vi "Average_ITP_curves.vi"(0 "I in":dbl[](array[numeric]), 1 "Averaged P(T) In":dbl[][](array[numeric]), 2 "Counter":i8, 5 "Averaged I(T) In":dbl[][](array[numeric]), 7 "t in":dbl[](array[numeric]), 9 "T in":dbl[](array[numeric]), 11 "Averaged dt in":dbl[][](array[numeric]), 12 "Up/Down":bool, 13 "Sample area(mm^2)":dbl, 14 "T array":dbl[](array[numeric])) -> (4 "Averaged I(B) out":dbl[][](array[numeric]), 6 "Averaged dt Out":dbl[][](array[numeric]), 8 "Averaged P(T) Out":dbl[][](array[numeric]))   [LabVIEW 2015]
uses:
  <vilib>/Analysis/baseanly.llb/Mean (DBL).vi
  <vilib>/Analysis/NI_AALBase.lvlib
  <vilib>/gmath/NI_Gmath.lvlib
panel:
  out "yi":dbl[](array[numeric]) format="%_6g"
  out "Down":cluster{"B array":dbl[], dbl[]}(graph)
  out "XY Graph 2":cluster{"B in":dbl[], "I in":dbl[]}(graph)
  out "Up":cluster{"B array":dbl[], dbl[]}(graph)
  out "subarray 2":dbl[](array[numeric])
  out "subarray":dbl[](array[numeric])
  out "Sorted array":dbl[][](array[numeric]) format="%.5f"
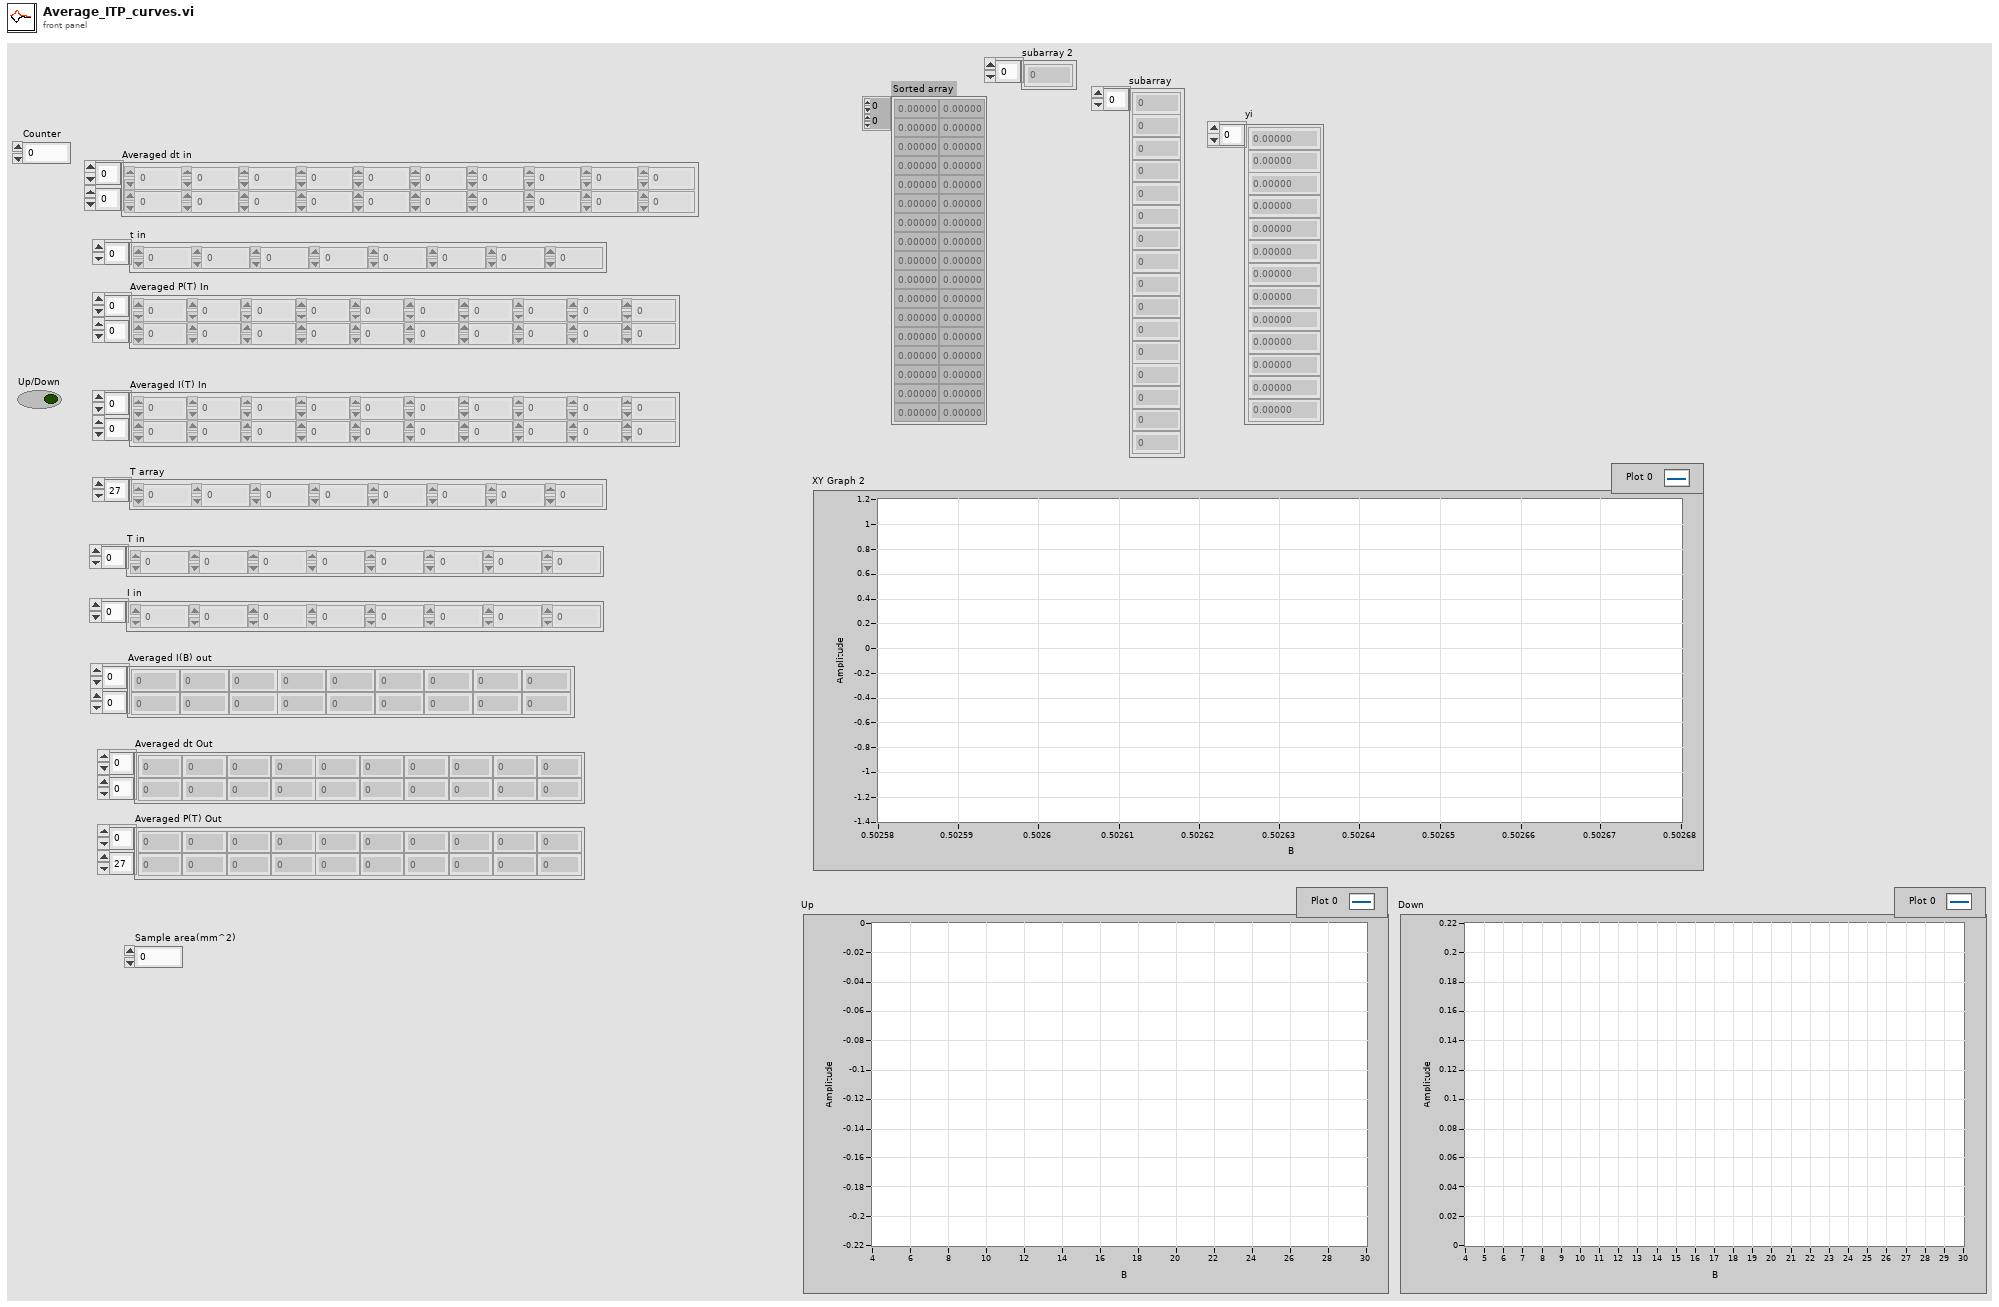
[diagram p1: front panel]
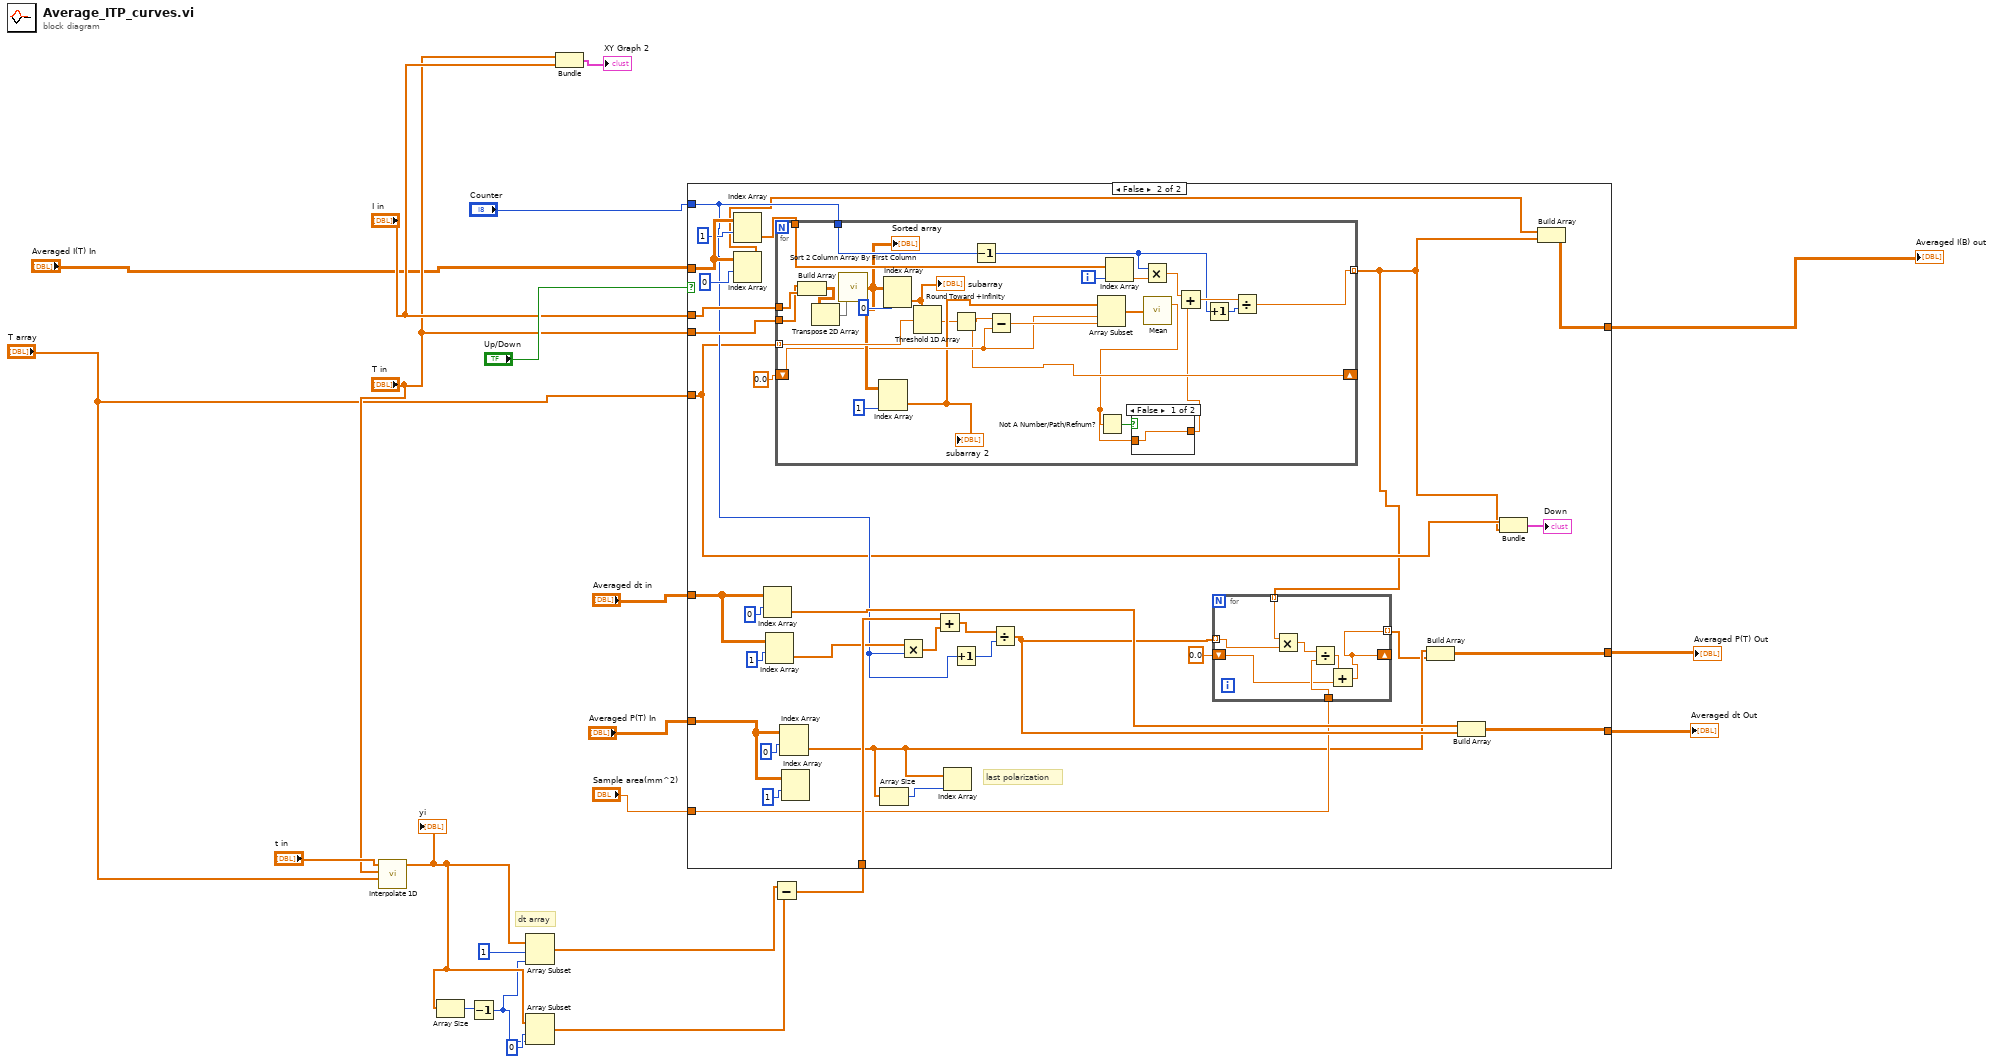
[diagram p0: block diagram]
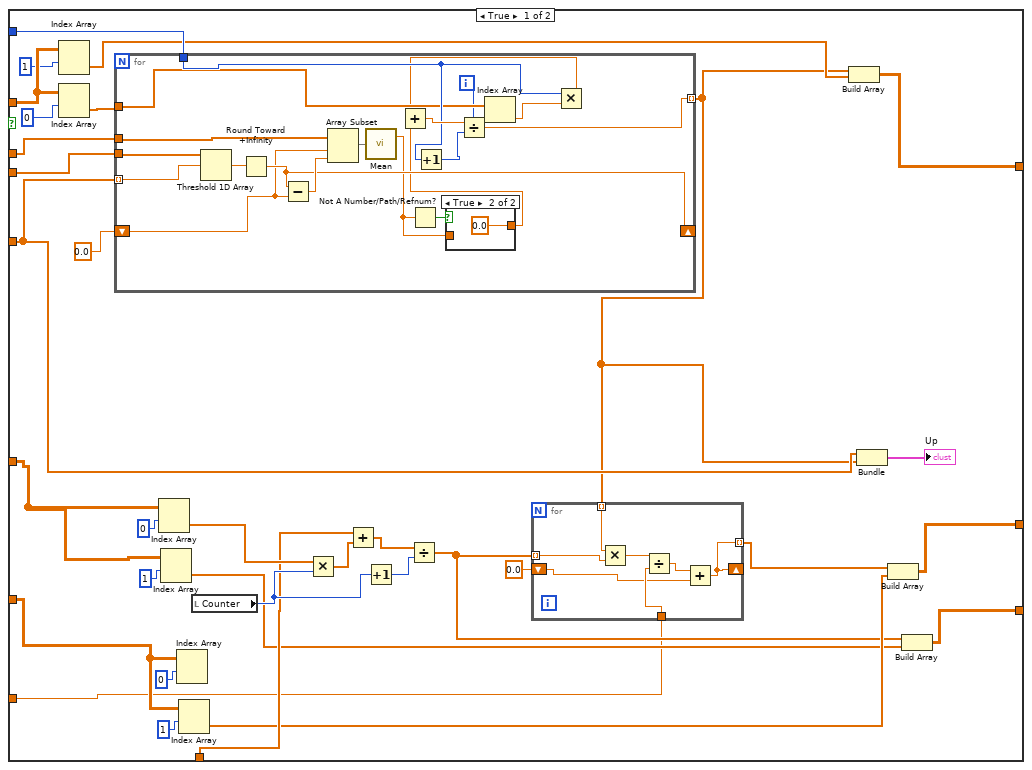
[diagram p2: hidden frame]
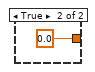
[diagram p4: hidden frame]
diagram:
  # "dt array"
  n1 = call <vilib>:"Interpolate 1D.vi"("xi"="T array", "X"="T in", "Y"="t in") -> ("yi"=w7:dbl[])  [unwired: 6 in, 2 out]
  "yi" <- w7
  n2 = Array Size(array=w7) -> (size(s)=w10:i32)
  n3 = Decrement(x=w10) -> (x-1=w3:i32)
  n4 = Array Subset(array=w7, index=1, length=w3) -> (w6:dbl[])
  n5 = Array Subset(array=w7, index=0, length=w3) -> (w5:dbl[])
  n6 = Bundle("T in"="T in", "I in"="I in") -> (→"XY Graph 2":cluster{"T in":dbl[], "I in":dbl[]})  [unwired: 1 in]
  n7 = Subtract(x=w6, y=w5) -> (x-y=w13:dbl[])
  n8 = case shown="False" "Up/Down" {
    tunnel: "Averaged I(T) In" -> [w51 w114]
    tunnel: "I in" -> [w53 w115]
    tunnel: "T in" -> [w34 w99]
    tunnel: "Counter" -> [w52 w87]
    tunnel: "T array" -> [w25 w86]
    tunnel: [w50 w88] -> w22
    tunnel: "Averaged dt in" -> [w41 w106]
    tunnel: "Averaged P(T) In" -> [w40 w105]
    tunnel: w13 -> [w39 w104]
    tunnel: [w37 w103] -> w17
    tunnel: [w35 w100] -> w16
    tunnel: "Sample area(mm^2)" -> [w26 w93]
    frame True {
      n9 = Index Array(array=w51, index (row)=1 ("disabled index (col)")) -> (element=w24:dbl[])  [unwired: 1 in]
      n10 = Index Array(array=w51, index (row)=0 ("disabled index (col)")) -> (element=w55:dbl[])  [unwired: 1 in]
      n11 = for {
        tunnel: w55 -> [w74]
        tunnel: w25 -> [w64] mode=indexing
        tunnel: w34 -> [w81]
        shift-right: [w69] -> _
        shift-left: 0.0 -> [w68]
        tunnel: w53 -> [w80]
        tunnel: w52 -> [w76]
        tunnel: [w75] -> w23 mode=indexing
        i -> [w73]
        n12 = Threshold 1D Array(2:w64, 3:w81) -> (0:w70:dbl)  [unwired: 1 in]
        n13 = Round Toward +Infinity(x=w70) -> (ceil(x): smallest int >= x=w69:dbl)
        n14 = Subtract(x=w69, y=w68) -> (x-y=w79:dbl)
        n15 = Array Subset(array=w80, index=w68, length=w79) -> (w71:dbl[])
        n16 = call-poly <vilib>:"Mean.vi"("X"=w71) -> ("mean"=w66:dbl)  [unwired: 1 out]
        n17 = Not A Number/Path/Refnum?(number/path/refnum=w66) -> (NaN/Path/Refnum?=w67:bool)
        n18 = Increment(x=w76) -> (x+1=w77:i8)
        n19 = case shown="True" w67 {
          tunnel: [w82 0.0] -> w65
          tunnel: w66 -> [w82 _]
          frame False {
          }
          frame True {
          }
        }
        n20 = Index Array(array=w74, index=w73) -> (element=w72:dbl)
        n21 = Multiply(x=w76, y=w72) -> (x*y=w63:dbl)
        n22 = Add(x=w63, y=w65) -> (x+y=w78:dbl)
        n23 = Divide(x=w78, y=w77) -> (x/y=w75:dbl)
      }
      n24 = Index Array(array=w41, index (row)=0 ("disabled index (col)")) -> (element=w42:dbl[])  [unwired: 1 in]
      n25 = Index Array(array=w41, index (row)=1 ("disabled index (col)")) -> (element=w36:dbl[])  [unwired: 1 in]
      n26 = Index Array(array=w40, index (row)=0 ("disabled index (col)")) -> ()  [unwired: 1 in, 1 out]
      n27 = Index Array(array=w40, index (row)=1 ("disabled index (col)")) -> (element=w38:dbl[])  [unwired: 1 in]
      n28 = local read "Counter"() -> (w44:i8)
      n29 = Multiply(x=w42, y=w44) -> (x*y=w43:dbl[])
      n30 = Add(x=w39, y=w43) -> (x+y=w45:dbl[])
      n31 = Increment(x=w44) -> (x+1=w46:i8)
      n32 = Divide(x=w45, y=w46) -> (x/y=w29:dbl[])
      n33 = for {
        shift-right: [w57] -> _
        shift-left: 0.0 -> [w56]
        tunnel: [w57] -> w27 mode=indexing
        tunnel: w23 -> [w62] mode=indexing
        tunnel: w29 -> [w61] mode=indexing
        tunnel: w26 -> [w60]
        n34 = Multiply(x=w62, y=w61) -> (x*y=w59:dbl)
        n35 = Divide(x=w59, y=w60) -> (x/y=w58:dbl)
        n36 = Add(x=w58, y=w56) -> (x+y=w57:dbl)
      }
      n37 = Build Array(w23, w24) -> (w50:dbl[][])
      n38 = Bundle("T array"=w25, w23) -> (→"Up":cluster{"T array":dbl[], dbl[]})  [unwired: 1 in]
      n39 = Build Array(w27, w38) -> (w37:dbl[][])
      n40 = Build Array(w29, w36) -> (w35:dbl[][])
    }
    frame False {
      # "last polarization"
      n41 = Index Array(array=w114, index (row)=1 ("disabled index (col)")) -> (element=w113:dbl[])  [unwired: 1 in]
      n42 = Index Array(array=w114, index (row)=0 ("disabled index (col)")) -> (element=w85:dbl[])  [unwired: 1 in]
      n43 = Index Array(array=w106, index (row)=0 ("disabled index (col)")) -> (element=w101:dbl[])  [unwired: 1 in]
      n44 = Index Array(array=w106, index (row)=1 ("disabled index (col)")) -> (element=w102:dbl[])  [unwired: 1 in]
      n45 = for {
        tunnel: w113 -> [w144]
        tunnel: w86 -> [w150] mode=indexing
        tunnel: w99 -> [w139]
        shift-right: [w129] -> _
        shift-left: 0.0 -> [w132]
        tunnel: w115 -> [w140]
        tunnel: w87 -> [w145]
        tunnel: [w124] -> w84 mode=indexing
        i -> [w143]
        n46 = Build Array(w139, w140) -> (w134:dbl[][])
        n47 = Transpose 2D Array(2D array=w134) -> (transposed array=w133:dbl[][])
        n48 = call "Sort 2 Column Array By First Column.vi"("2D array to sort"=w133) -> ("Sorted array"=w136:dbl[][])
        "Sorted array" <- w136
        n49 = Index Array(array=w136, index (col)=1 ("disabled index (col)")) -> (element=w131:dbl[])  [unwired: 1 in]
        "subarray 2" <- w131
        n50 = Index Array(array=w136, index (col)=0 ("disabled index (col)")) -> (element=w138:dbl[])  [unwired: 1 in]
        "subarray" <- w138
        n51 = Threshold 1D Array(2:w150, 3:w138) -> (0:w130:dbl)  [unwired: 1 in]
        n52 = Round Toward +Infinity(x=w130) -> (ceil(x): smallest int >= x=w129:dbl)
        n53 = Decrement(x=w145) -> (x-1=w125:i8)
        n54 = Subtract(x=w129, y=w132) -> (x-y=w149:dbl)
        n55 = Array Subset(array=w131, index=w132, length=w149) -> (w141:dbl[])
        n56 = Index Array(array=w144, index=w143) -> (element=w142:dbl)
        n57 = Multiply(x=w125, y=w142) -> (x*y=w148:dbl)
        n58 = call-poly <vilib>:"Mean.vi"("X"=w141) -> ("mean"=w127:dbl)  [unwired: 1 out]
        n59 = Not A Number/Path/Refnum?(number/path/refnum=w127) -> (NaN/Path/Refnum?=w128:bool)
        n60 = case shown="False" w128 {
          tunnel: [w151 0.0] -> w126
          tunnel: w127 -> [w151 _]
          frame False {
          }
          frame True {
          }
        }
        n61 = Add(x=w148, y=w126) -> (x+y=w147:dbl)
        n62 = Increment(x=w125) -> (x+1=w146:i8)
        n63 = Divide(x=w147, y=w146) -> (x/y=w124:dbl)
      }
      n64 = Index Array(array=w105, index (row)=0 ("disabled index (col)")) -> (element=w92:dbl[])  [unwired: 1 in]
      n65 = Index Array(array=w105, index (row)=1 ("disabled index (col)")) -> ()  [unwired: 1 in, 1 out]
      n66 = Array Size(array=w92) -> (size(s)=w91:i32)
      n67 = Multiply(x=w102, y=w87) -> (x*y=w107:dbl[])
      n68 = Add(x=w104, y=w107) -> (x+y=w108:dbl[])
      n69 = Index Array(array=w92, index=w91) -> ()  [unwired: 1 out]
      n70 = Increment(x=w87) -> (x+1=w109:i8)
      n71 = Divide(x=w108, y=w109) -> (x/y=w94:dbl[])
      n72 = for {
        tunnel: w94 -> [w122] mode=indexing
        tunnel: w84 -> [w121] mode=indexing
        shift-right: [w119] -> _
        shift-left: 0.0 -> [w117]
        tunnel: [w119] -> w89 mode=indexing
        tunnel: w93 -> [w118]
        n73 = Multiply(x=w121, y=w122) -> (x*y=w123:dbl)
        n74 = Divide(x=w123, y=w118) -> (x/y=w120:dbl)
        n75 = Add(x=w120, y=w117) -> (x+y=w119:dbl)
      }
      n76 = Build Array(w92, w89) -> (w103:dbl[][])
      n77 = Build Array(w101, w94) -> (w100:dbl[][])
      n78 = Bundle("T array"=w86, w84) -> (→"Down":cluster{"T array":dbl[], dbl[]})  [unwired: 1 in]
      n79 = Build Array(w85, w84) -> (w88:dbl[][])
    }
  }
  "Averaged I(B) out" <- w22
  "Averaged P(T) Out" <- w17
  "Averaged dt Out" <- w16
